vi "maptests.vi"() -> ()   [LabVIEW 2020]
uses:
  3-lorentzian-parameters.ctl
panel:
  in  "parameters":T1={"κ0"=1.0234079529926423e-07, "τC"=0.013647490503661961, "τN"=4.235643214853134e-05, "τS"=0.13437466196040418, "T1"=0.009762017848695768, "ζ"=0.00391493831404709} {"ζ" min=0.0 max=0.3 step=1e-06 scale=1e-05..1000.0 scale format="%#_3p"; "T1" min=0.0 max=0.3 step=1e-06 scale=0.0001..10.0 scale format="%#_3p"; "τS" min=0.0 max=0.3 step=1e-06 scale=0.0001..10.0 scale format="%#_3p"; "τN" min=0.0 max=0.3 step=1e-06 scale=1e-06..10.0 scale format="%#_3p"; "τC" min=0.0 max=0.3 step=1e-06 scale=0.0001..10.0 scale format="%#_3p"; "κ0" min=0.0 max=0.3 step=1e-12 scale=1e-10..1e-06 scale format="%#_3p"}
  in  "parameters":enum32{"Page 1"}(tab)
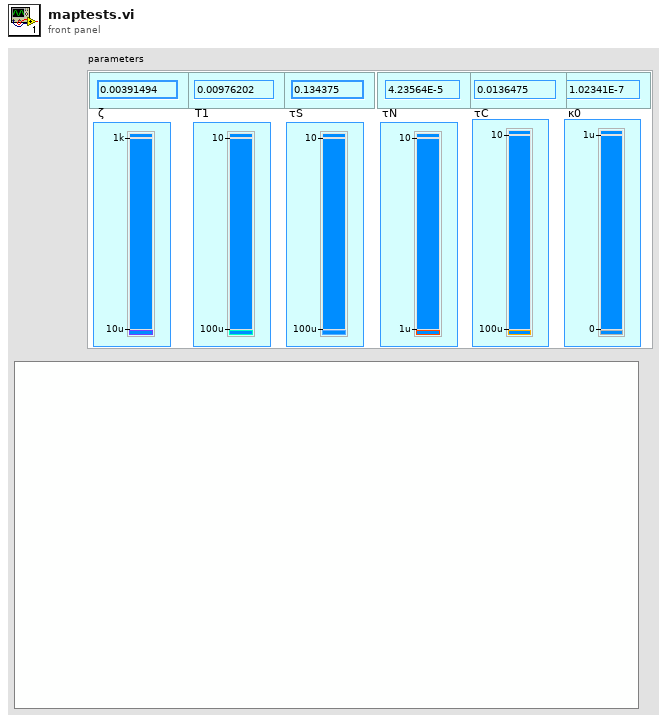
[diagram p1: front panel]
types:
  T1 = cluster{"κ0":dbl, "τC":dbl, "τN":dbl, "τS":dbl, "T1":dbl, "ζ":dbl}
  T2 = typedef "3-lorentzian-parameters.ctl" = enum16{"ζ", "τ1", "τS", "τN", "τC", "κ0", "m1", "m2", "m3"}
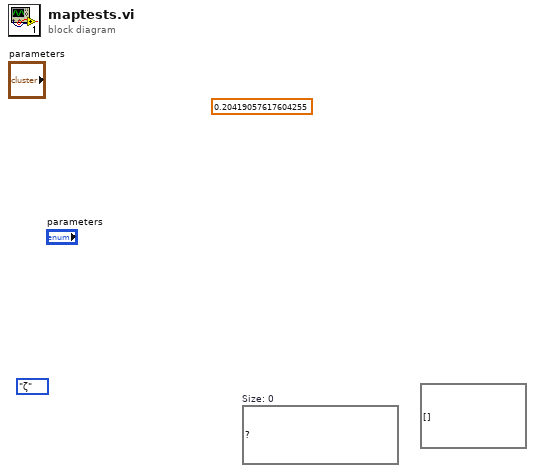
[diagram p0: block diagram]
diagram:
  (unwired) map{T2, dbl}[] []
  (unwired) 0.20419057617604255 ("ζ")
  (unwired) 3-lorentzian-parameters."ζ" ("Plost: sweep window")
  (unwired) map{T2, dbl} {}  # Size: 0
